vi "open.vi"(8 "error in (no error)":errorcluster, 11 "HamegHMPSupply in":refnum<class "HamegHMPSupply.lvclass">) -> (0 "error out":errorcluster, 3 "HamegHMPSupply out":refnum<class "HamegHMPSupply.lvclass">)   [LabVIEW 2009, in "Hardware.lvlib" / "Channels.lvlib" / "HamegHMPSupply.lvclass"]
uses:
  HamegHMPSupply.lvclass
  HamegHMPSupply.lvclass/HamegHMPSupply.ctl
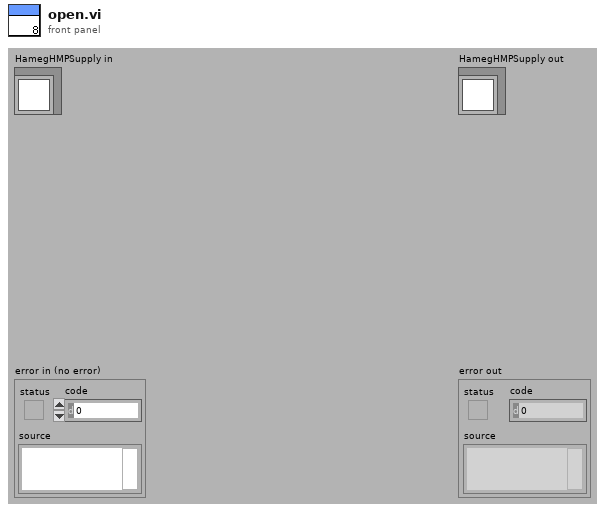
[diagram p1: front panel]
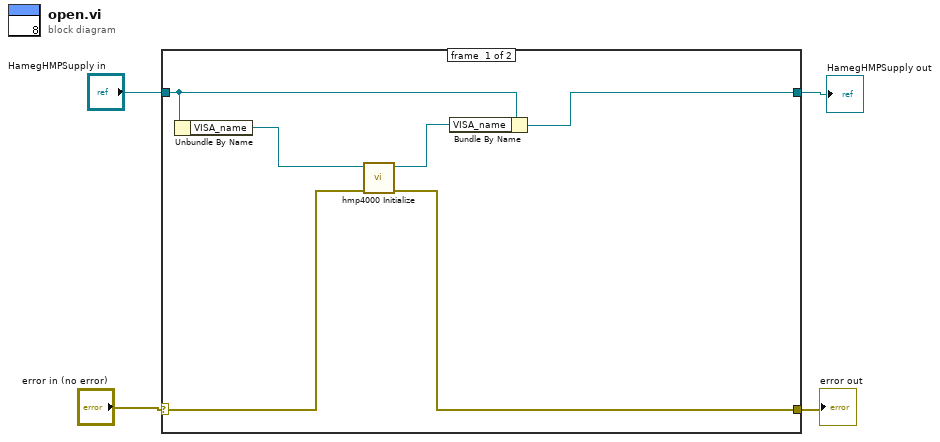
[diagram p0: block diagram]
diagram:
  n1 = case shown="No Error" "error in (no error)" {
    selector: "error in (no error)" -> [w9 w11]
    tunnel: [w5 w12] -> w3
    tunnel: "HamegHMPSupply in" -> [w6 w12]
    tunnel: [w7 w11] -> w1
    frame #0 {
      n2 = Unbundle By Name(w6) -> ("VISA_name"=w10:refnum<visa-resource-name>)
      n3 = call <instrlib>:"hmp4000 Initialize.vi"("error in (no error)"=w9, "VISA resource name"=w10) -> ("error out"=w7:errorcluster, "VISA resource name out"=w8:refnum<visa-resource-name>)  [unwired: 8 in]
      n4 = Bundle By Name(cluster=w6, "VISA_name"=w8) -> (w5:refnum<class "HamegHMPSupply.lvclass">)
    }
    frame #1 {
    }
  }
  "error out" <- w1
  "HamegHMPSupply out" <- w3
